vi "RunOperation.vi"(10 "Inputs":string[](array[string]), 11 "SecureRunVI in":refnum<class "SecureRunVI.lvclass">) -> (1 "Output/Failure":string, 2 "CLI Process Return Code":i32, 3 "SecureRunVI out":refnum<class "SecureRunVI.lvclass">)   [LabVIEW 2014, in "SecureRunVI.lvclass"]
doc: "Entry point for LabVIEWCLI."
uses:
  SecureRunVI.lvclass
  SecureRunVI.lvclass/SecureRunVI.ctl
  Utilities/BuildSecurity/BuildSecurity.lvlib
panel:
  in  "Format Error Output String":string="Error Code : %d\\nError Message : %s\\nAn error occurred while running the %s operation.\\n"
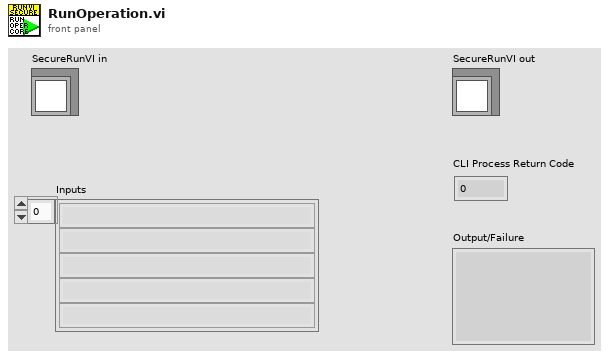
[diagram p1: front panel]
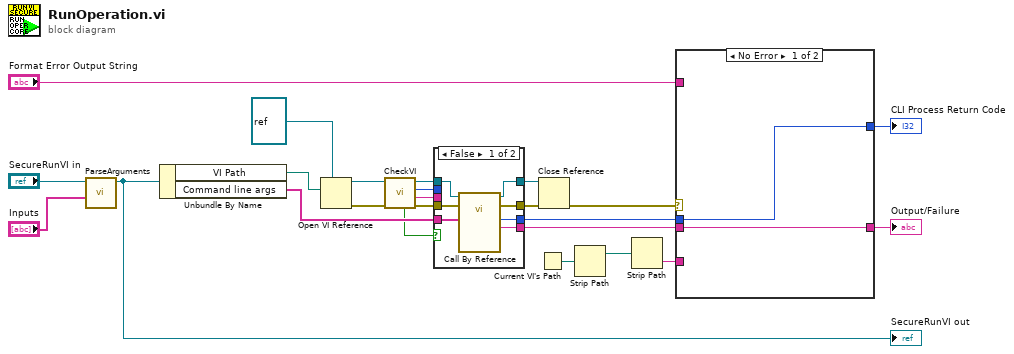
[diagram p0: block diagram]
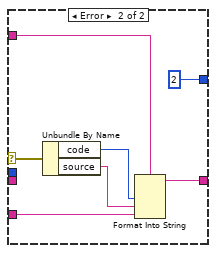
[diagram p3: hidden frame]
diagram:
  n1 = call "ParseArguments.vi"("Inputs"="Inputs", "SecureRunVI in"="SecureRunVI in") -> ("SecureRunVI out"=w6:refnum<class "SecureRunVI.lvclass">)  [unwired: 8 in, 1 out]
  "SecureRunVI out" <- w6
  n2 = Unbundle By Name(w6) -> ("VI Path"=w22:path, "Command line args"=w20:string[])
  n3 = Open VI Reference(type specifier VI Refnum (for type only)=refnum<vi> refnum, vi path=w22) -> (vi reference=w4:refnum<vi>, error out=w8:errorcluster)  [unwired: 4 in]
  n4 = call "CheckVI.vi"("error in (no error)"=w8, "VI Refnum"=w4) -> ("error out"=w7:errorcluster, "Output/Failure"=w1:string, "CLI Process Return Code"=w2:i32, "dup VI Refnum"=w5:refnum<vi>, "Reject?"=w3:bool)  [unwired: 5 in]
  n5 = case shown="False" w3 {
    tunnel: w20 -> [w31 _]
    tunnel: [w30 w35] -> w19
    tunnel: [w29 w34] -> w18
    tunnel: [w28 w33] -> w13
    tunnel: [w27 w32] -> w12
    tunnel: w7 -> [w26 w34]
    tunnel: w5 -> [w25 w35]
    tunnel: w2 -> [_ w33]
    tunnel: w1 -> [_ w32]
    frame False {
      n6 = call-by-ref "?"(reference=w25, error in=w26, "Inputs"=w31) -> (reference out=w30:refnum<vi>, error out=w29:errorcluster, "String"=w27:string, "Numeric"=w28:i32)  [unwired: 9 in]
    }
    frame True {
    }
  }
  n7 = Current VI's Path() -> (path=w16:path)
  n8 = Close Reference(reference=w19, error in (no error)=w18) -> (error out=w17:errorcluster)
  n9 = Strip Path(path=w16) -> (stripped path=w15:path)  [unwired: 1 out]
  n10 = Strip Path(path=w15) -> (name=w14:string)  [unwired: 1 out]
  n11 = case shown="No Error" w17 {
    selector: w17 -> [_ w41]
    tunnel: [w37 w38] -> w9
    tunnel: w12 -> [w37 _]
    tunnel: [w36 2 ("f")] -> w10
    tunnel: "Format Error Output String" -> [_ w43]
    tunnel: w14 -> [_ w42]
    tunnel: w13 -> [w36 _]
    frame No Error {
    }
    frame Error {
      n12 = Unbundle By Name(w41) -> ("code"=w40:i32, "source"=w39:string)
      n13 = Format Into String(format string=w43, w40, w39, w42) -> (resulting string=w38:string)  [unwired: 2 in, 1 out]
    }
  }
  "CLI Process Return Code" <- w10
  "Output/Failure" <- w9
